vi "Test_sqlite3Open_ErrorIfNotaPath.vi"(8 "error in (no error)":errorcluster, 11 "TestCase in":refnum<class "Test sqlite3.lvclass">) -> (0 "error out":errorcluster, 3 "TestCase out":refnum<class "Test sqlite3.lvclass">)   [LabVIEW 2020, in "Test sqlite3.lvclass"]
uses:
  Test sqlite3.lvclass
  externals/sqlite3/Source/sqlite3.lvclass/sqlite3.ctl
  <vilib>/Utility/error.llb/Error Cluster From Error Code.vi
  externals/sqlite3/Source/sqlite3.lvclass
  <vilib>/addons/_JKI Toolkits/VI Tester/TestCase.llb/TestCase.lvclass
  C:/Program Files/National Instruments/LabVIEW 2020/vi.lib/addons/_JKI Toolkits/VI Tester/TestCase.llb/TestCase.lvclass
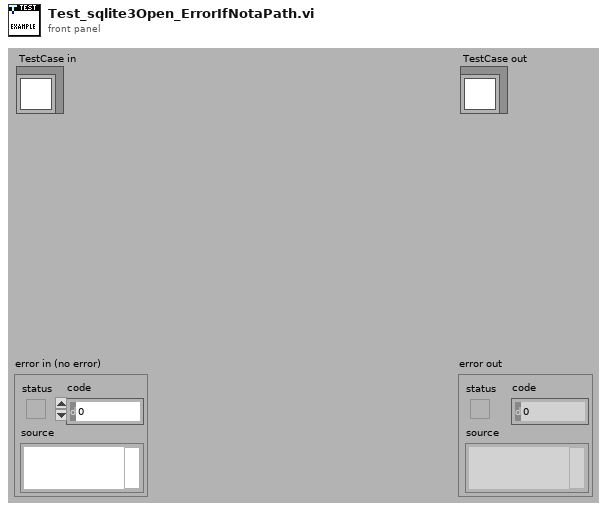
[diagram p1: front panel]
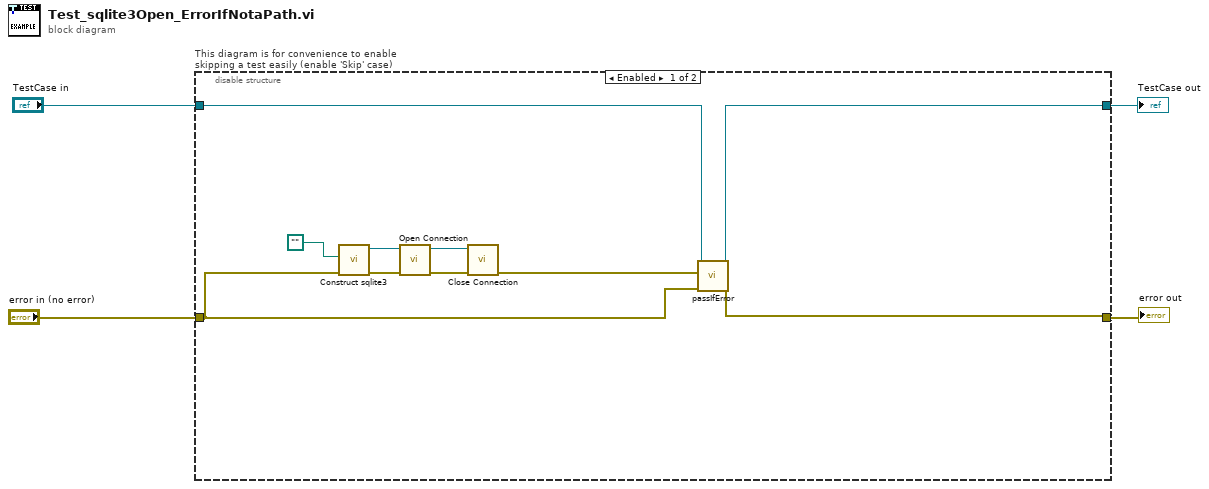
[diagram p0: block diagram]
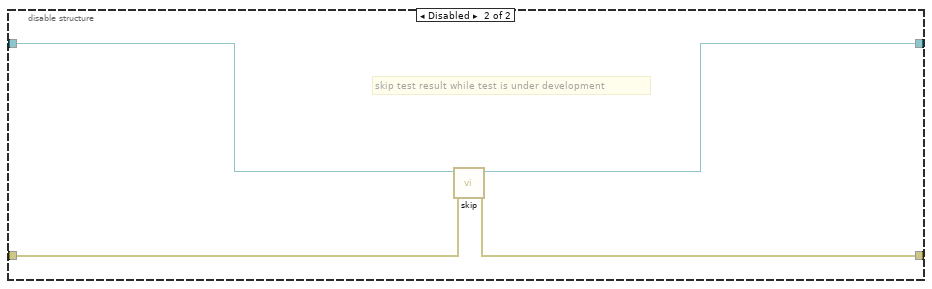
[diagram p2: hidden frame]
diagram:
  n1 = disable-structure "This diagram is for convenience to enable skipping a test easily (enable 'Skip' case)" shown="Enabled" {
    disable-tunnel: "TestCase in" -> [w14 w18]
    disable-tunnel: [w13 w16] -> w1
    disable-tunnel: [w12 w17] -> w3
    disable-tunnel: "error in (no error)" -> [w9 w15]
    frame Enabled {
      n2 = call "Construct sqlite3.vi"("error in (no error)"=w9, "DatabaseFilePath"=path "") -> ("error out"=w11:errorcluster, "sqlite3 out"=w8:refnum<class "sqlite3.lvclass">)  [unwired: 8 in]
      n3 = call-dynamic "Open Connection.vi"("error in (no error)"=w11, "sqlite in"=w8) -> ("error out"=w10:errorcluster, "sqlite out"=w7:refnum<class "sqlite3.lvclass">)  [unwired: 8 in]
      n4 = call-dynamic "Close Connection.vi"("error in (no error)"=w10, "sqlite in"=w7) -> ("error out"=w5:errorcluster)  [unwired: 8 in, 1 out]
      n5 = call-dynamic "passIfError.vi"("error in (no error)"=w9, "error"=w5, "TestCase in"=w14) -> ("error out"=w12:errorcluster, "TestCase out"=w13:refnum<class "Test sqlite3.lvclass">)  [unwired: 7 in]
    }
    frame Disabled {
      # "skip test result while test is under development"
      n6 = call <vilib>:"skip.vi"("error in (no error)"=w15, "TestCase in"=w18) -> ("error out"=w17:errorcluster, "TestCase out"=w16:refnum<class "Test sqlite3.lvclass">)  [unwired: 8 in]
    }
  }
  "error out" <- w3
  "TestCase out" <- w1
